vi "thermometer .vi"() -> ()   [LabVIEW 2019]
panel:
  in  "stop 2":bool
  in  "Numeric 2":dbl
  out "Thermometer 2":dbl(slide) scale=0.0..100.0
  in  "Thermometer":dbl(slide) scale=0.0..100.0
  in  "Numeric":dbl
  in  "stop":bool
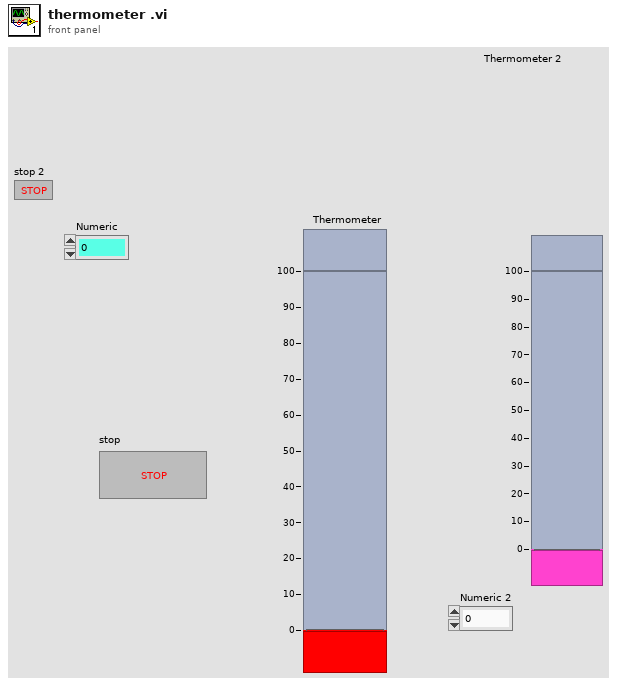
[diagram p1: front panel]
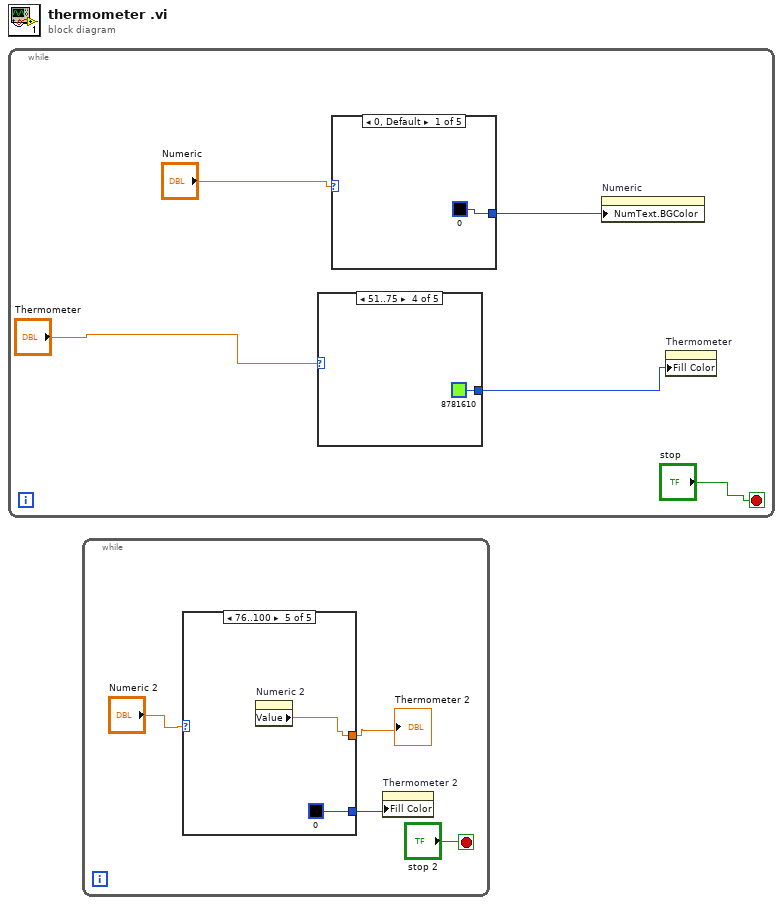
[diagram p0: block diagram]
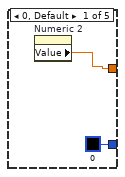
[diagram p2: hidden frame]
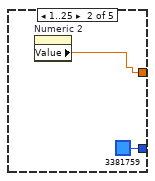
[diagram p3: hidden frame]
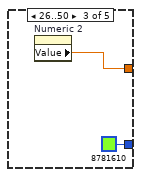
[diagram p4: hidden frame]
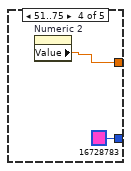
[diagram p5: hidden frame]
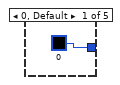
[diagram p6: hidden frame]
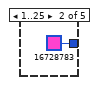
[diagram p7: hidden frame]
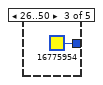
[diagram p8: hidden frame]
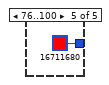
[diagram p9: hidden frame]
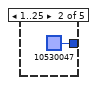
[diagram p10: hidden frame]
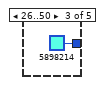
[diagram p11: hidden frame]
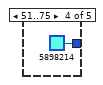
[diagram p12: hidden frame]
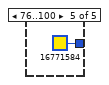
[diagram p13: hidden frame]
diagram:
  n1 = while {
    stop <- "stop" stop-if-true
    n2 = case shown="51..75" "Thermometer" {
      tunnel: [u32 0 ("Numeric Text.Text Colors:BG Color") u32 16728783 ("Numeric Text.Text Colors:BG Color") u32 16775954 ("Numeric Text.Text Colors:BG Color") u32 8781610 ("Numeric Text.Text Colors:BG Color") u32 16711680 ("Numeric Text.Text Colors:BG Color")] -> w1
      frame 0, Default {
      }
      frame 1..25 {
      }
      frame 26..50 {
      }
      frame 51..75 {
      }
      frame 76..100 {
      }
    }
    n3 = case shown="0, Default" "Numeric" {
      tunnel: [u32 0 ("Numeric Text.Text Colors:BG Color") u32 10530047 ("Numeric Text.Text Colors:BG Color") u32 5898214 ("Numeric Text.Text Colors:BG Color") u32 5898214 ("Numeric Text.Text Colors:BG Color") u32 16771584 ("Numeric Text.Text Colors:BG Color")] -> w4
      frame 0, Default {
      }
      frame 1..25 {
      }
      frame 26..50 {
      }
      frame 51..75 {
      }
      frame 76..100 {
      }
    }
    n4 = property on="Numeric" class="DigNum (strict)"("NumText.BGColor"=w4) -> ()  [unwired: 2 in, 2 out]
    n5 = property on="Thermometer" class="Slide (strict)"("Fill Color"=w1) -> ()  [unwired: 2 in, 2 out]
  }
  n6 = while {
    stop <- "stop 2" stop-if-true
    n7 = case shown="76..100" "Numeric 2" {
      tunnel: [u32 0 ("Fill Color") u32 3381759 ("Fill Color") u32 8781610 ("Fill Color") u32 16728783 ("Fill Color") u32 0 ("Fill Color")] -> w18
      tunnel: [w20 w22 w24 w26 w28] -> w16
      frame 0, Default {
        n8 = property on="Numeric 2" class="DigNum (strict)"() -> ("Value"=w20:dbl)  [unwired: 2 in, 2 out]
      }
      frame 1..25 {
        n9 = property on="Numeric 2" class="DigNum (strict)"() -> ("Value"=w22:dbl)  [unwired: 2 in, 2 out]
      }
      frame 26..50 {
        n10 = property on="Numeric 2" class="DigNum (strict)"() -> ("Value"=w24:dbl)  [unwired: 2 in, 2 out]
      }
      frame 51..75 {
        n11 = property on="Numeric 2" class="DigNum (strict)"() -> ("Value"=w26:dbl)  [unwired: 2 in, 2 out]
      }
      frame 76..100 {
        n12 = property on="Numeric 2" class="DigNum (strict)"() -> ("Value"=w28:dbl)  [unwired: 2 in, 2 out]
      }
    }
    "Thermometer 2" <- w16
    n13 = property on="Thermometer 2" class="Slide (strict)"("Fill Color"=w18) -> ()  [unwired: 2 in, 2 out]
  }
